vi "Config.vi"() -> ()   [LabVIEW 2020]
uses:
  Global_Variable/Global.vi
  Global_Variable/A180648.vi
  <vilib>/Utility/config.llb/NI_LVConfig.lvlib
  Libraries/S7/S7.lvlib
panel:
  in  "试验项目":cluster{"拉轴":bool, "卡簧":bool}
  in  "产品型号":string(combo)
  in  "删除":bool
  in  "确定":bool
  in  "添加":bool
  in  "退出":bool
  in  "更新":bool
  in  "选项卡控件":enum32{"产品参数"}(tab)
  in  "结果判定参数":string[][](table)=[["mm"], ["KN"], ["KN"], ["KN"], [""], [""], [""], [""], [""], [""], [""], [""]]
  in  "判定框参数":string[][](table)=[["mm"], ["KN"], ["mm"], ["KN"]]
  in  "坐标轴参数":string[][](table)=[[""], ["°/S"], ["°"], ["Nm"]]
  # "上转向轴组件压装"
types:
  T1 = typedef "NI_LVConfig.lvlib/Config Data RefNum.ctl" = refnum<k1>
  T2 = cluster{"[0]":cluster{string, dbl, dbl}, "[1]":cluster{string, dbl, dbl}, "[2]":cluster{string, dbl, dbl}, "[3]":cluster{string, dbl, dbl}}
  T3 = cluster{"第一段位移":cluster{"单位":string, "下限":dbl, "上限":dbl}, "第一段压力":cluster{"单位":string, "下限":dbl, "上限":dbl}, "第二段位移":cluster{"单位":string, "下限":dbl, "上限":dbl}, "第二段压力":cluster{"单位":string, "下限":dbl, "上限":dbl}}
  T4 = cluster{"[0]":cluster{string, dbl, dbl}, "[1]":cluster{string, dbl, dbl}, "[2]":cluster{string, dbl, dbl}, "[3]":cluster{string, dbl, dbl}, "[4]":cluster{string, dbl, dbl}}
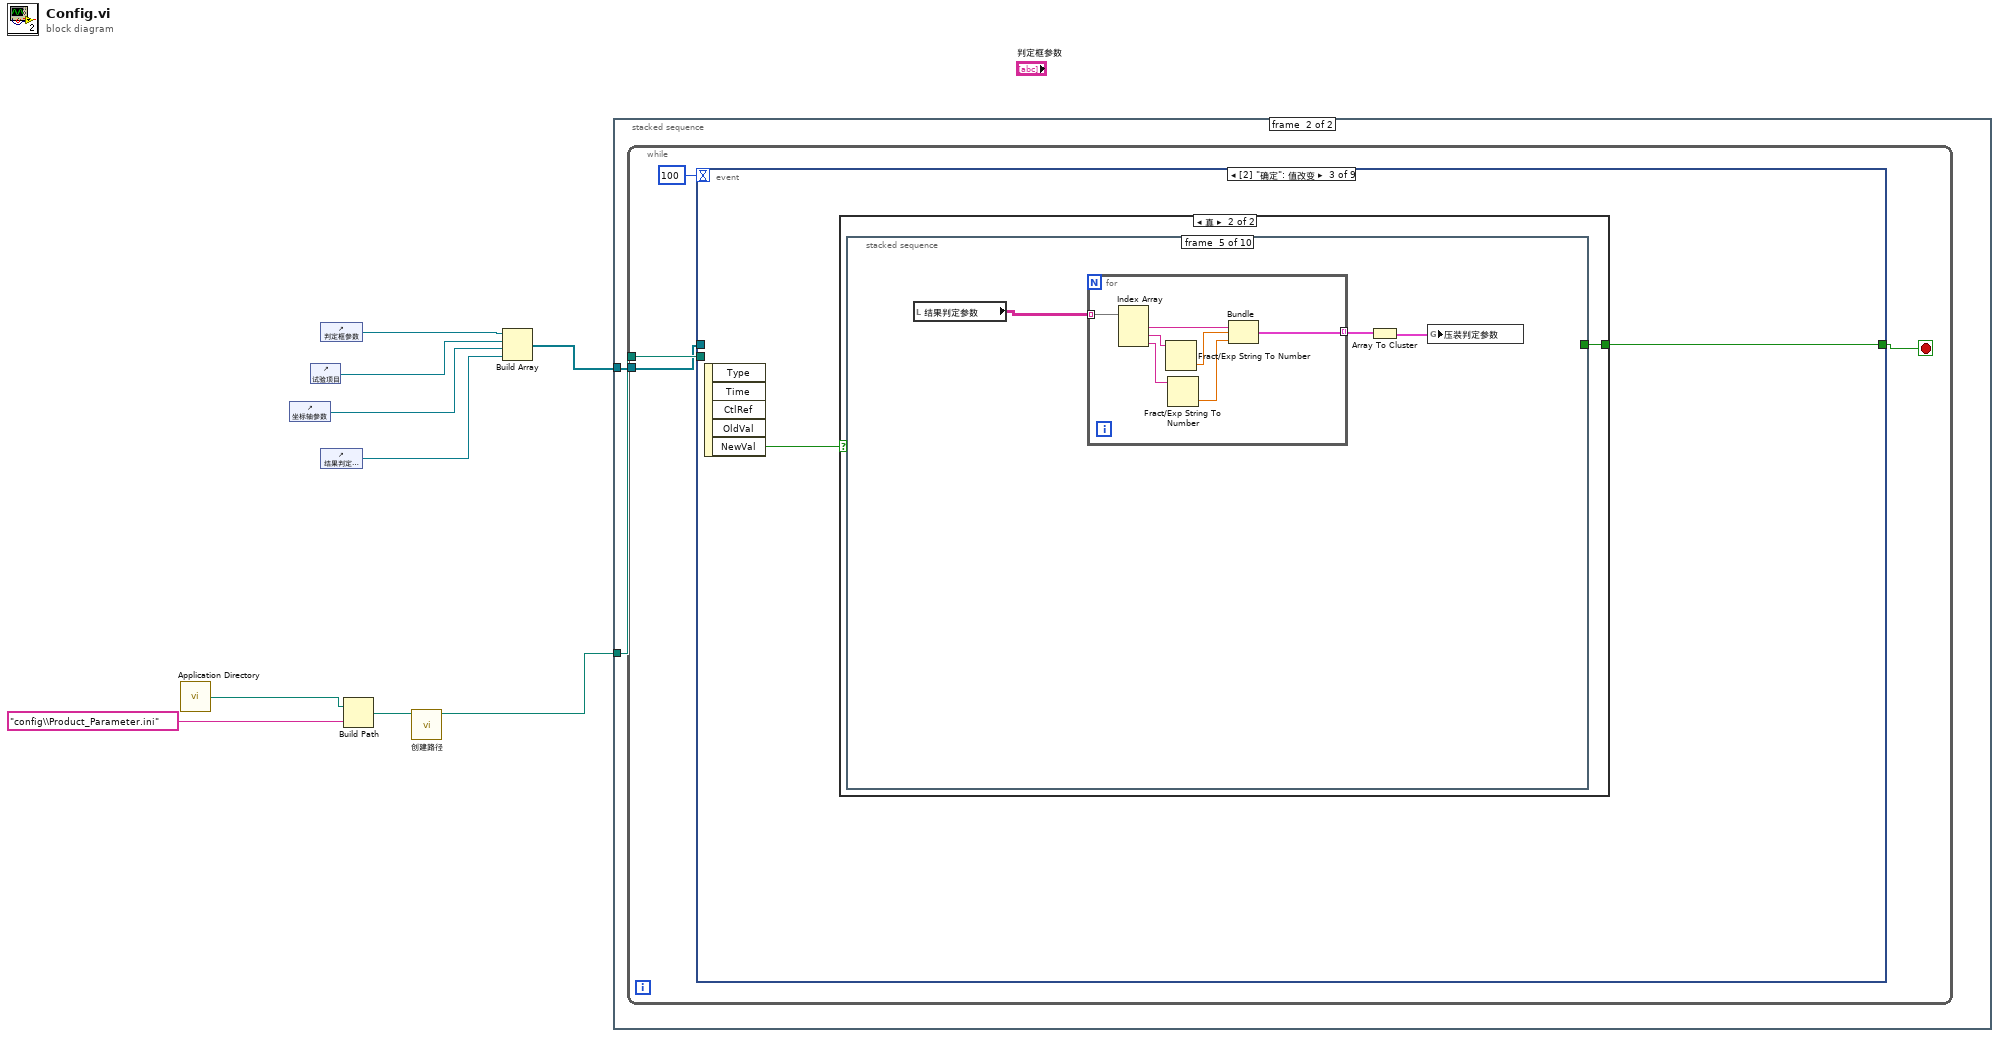
[diagram p0: block diagram]
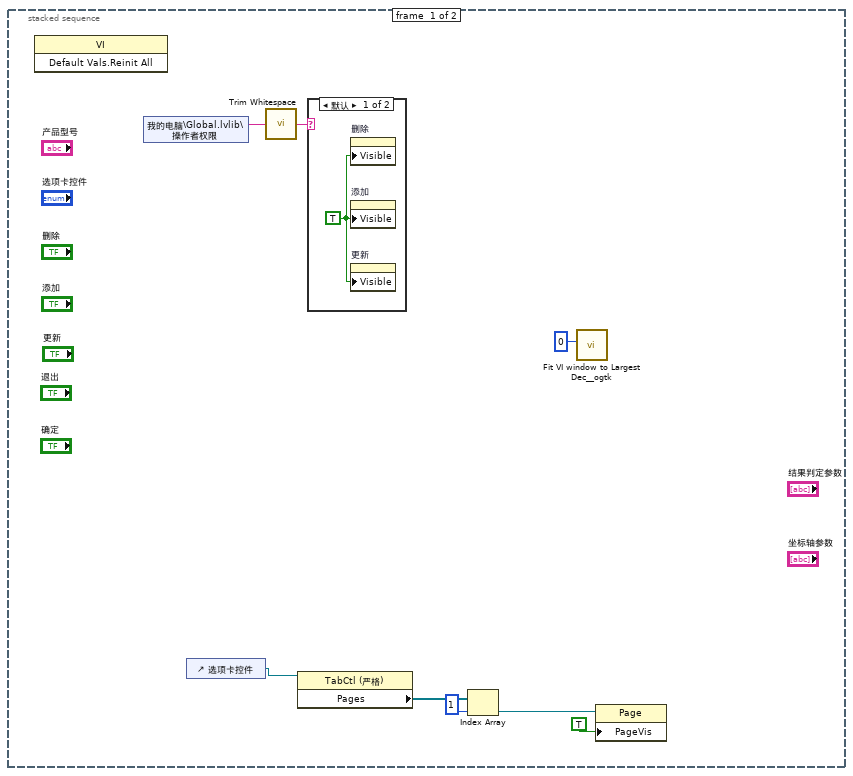
[diagram p2: hidden frame]
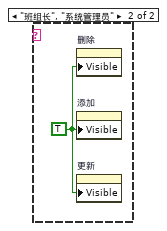
[diagram p3: hidden frame]
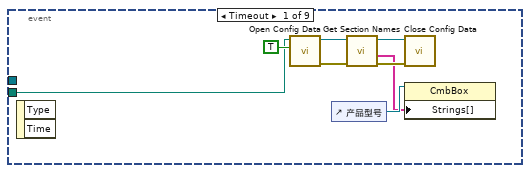
[diagram p4: hidden frame]
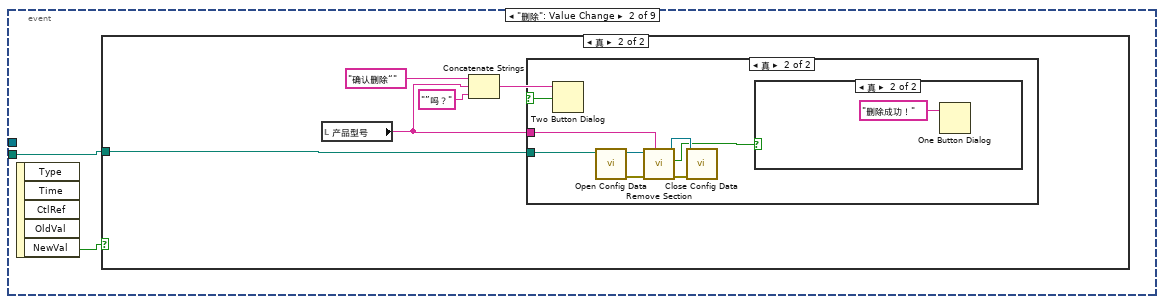
[diagram p5: hidden frame]
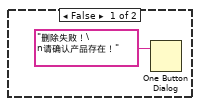
[diagram p8: hidden frame]
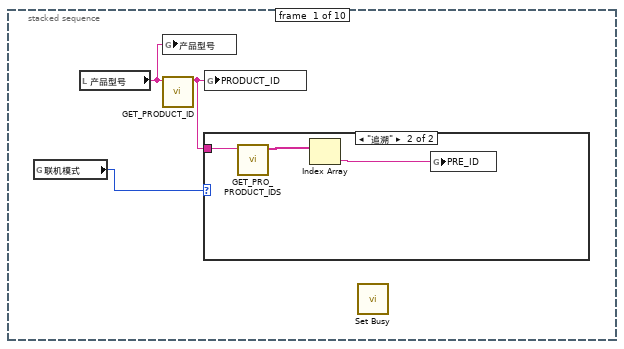
[diagram p10: hidden frame]
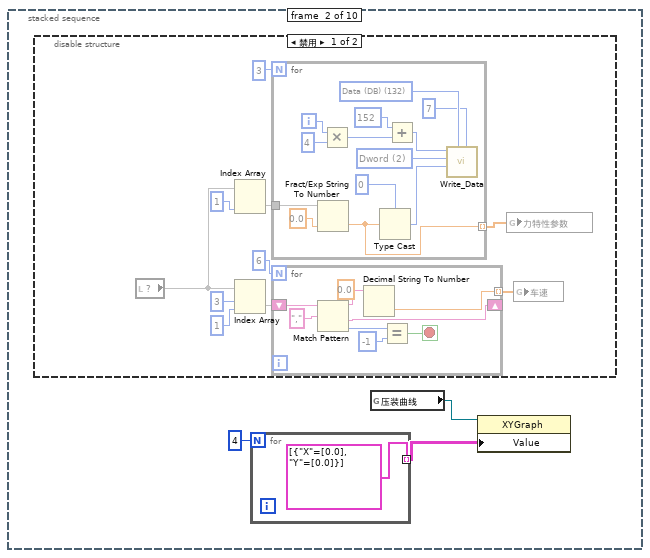
[diagram p12: hidden frame]
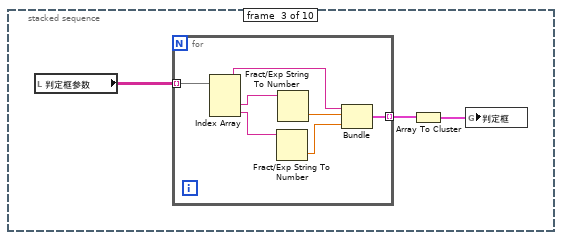
[diagram p14: hidden frame]
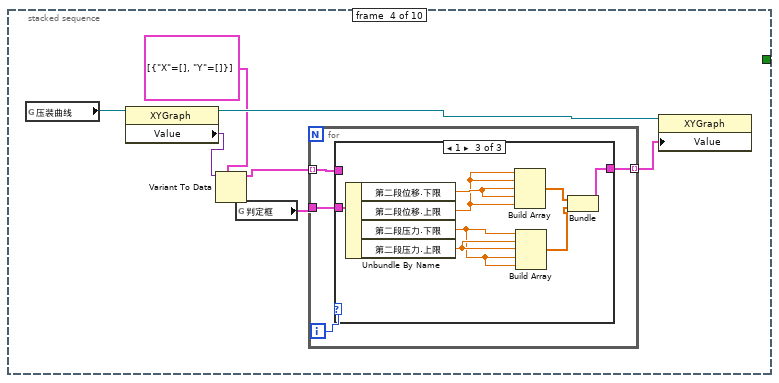
[diagram p15: hidden frame]
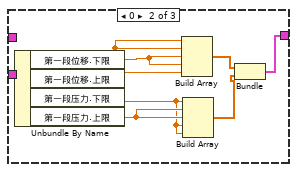
[diagram p17: hidden frame]
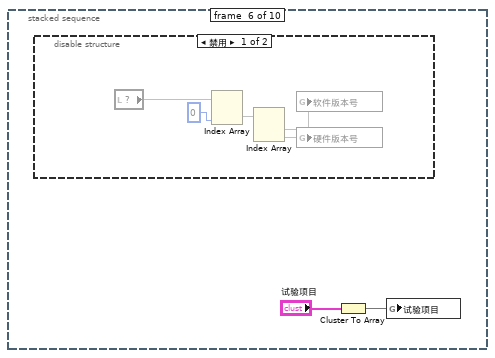
[diagram p18: hidden frame]
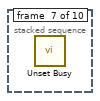
[diagram p20: hidden frame]
diagram:
  n1 = call <vilib>:"Application Directory.vi"() -> ("Application Directory"=w8:path)
  n2 = control-ref of="坐标轴参数"() -> (w3:refnum<vi>)
  n3 = control-ref of="试验项目"() -> (w4:refnum<vi>)
  n4 = control-ref of="判定框参数"() -> (w1:refnum<vi>)
  n5 = control-ref of="结果判定参数"() -> (w2:refnum<vi>)
  n6 = Build Path(base path=w8, name or relative path="config\\Product_Parameter.ini" ("名称或相对路径")) -> (appended path=w6:path)
  n7 = call "创建路径.vi"("path"=w6) -> ("path out"=w5:path)  [unwired: 9 in, 1 out]
  n8 = Build Array(w1, w4, w3, w2) -> (w9:refnum<vi>[])
  n9 = stacked-sequence {
    tunnel: w9 -> [_ w21]
    tunnel: w5 -> [_ w20]
    frame #0 {
      n10 = invoke class="VI" method="Default Vals.Reinit All"() -> ()  [unwired: 3 in, 3 out]
      n11 = shared-variable "我的电脑\\Global.lvlib\\操作者权限"() -> (w17:string)  [unwired: 1 in, 1 out]
      n12 = control-ref of="选项卡控件"() -> (w14:refnum<vi>)
      n13 = call <vilib>:"Trim Whitespace.vi"("string"=w17) -> ("trimmed string"=w16:string)  [unwired: 1 in]
      n14 = property class="TabCtl (严格)"(reference=w14) -> ("Pages"=w13:refnum<vi>[])  [unwired: 1 in, 2 out]
      n15 = case shown="默认" w16 {
        frame Default {
          w18 = TRUE ("可见")
          n16 = property on="删除" class="Bool (严格)"("Visible"=w18) -> ()  [unwired: 2 in, 2 out]
          n17 = property on="添加" class="Bool (严格)"("Visible"=w18) -> ()  [unwired: 2 in, 2 out]
          n18 = property on="更新" class="Bool (严格)"("Visible"=w18) -> ()  [unwired: 2 in, 2 out]
        }
        frame "班组长", "系统管理员" {
          w19 = TRUE ("可见")
          n19 = property on="删除" class="Bool (严格)"("Visible"=w19) -> ()  [unwired: 2 in, 2 out]
          n20 = property on="添加" class="Bool (严格)"("Visible"=w19) -> ()  [unwired: 2 in, 2 out]
          n21 = property on="更新" class="Bool (严格)"("Visible"=w19) -> ()  [unwired: 2 in, 2 out]
        }
      }
      n22 = Index Array(array=w13, index=1 ("索引")) -> (element=w12:refnum<vi>)
      n23 = call <userlib>:"Fit VI window to Largest Dec__ogtk.vi"("border spacing (2 px)"=0) -> ()  [unwired: 5 in, 2 out]
      n24 = property class="Page"(reference=w12, "PageVis"=TRUE ("选项卡可见")) -> ()  [unwired: 1 in, 2 out]
    }
    frame #1 {
      n25 = while {
        tunnel: w20 -> [w25]
        tunnel: w21 -> [w23]
        stop <- w24 stop-if-true
        n26 = event shown="[2] \"确定\": 值改变" {
          selector: _ -> [_ _ _ _ _ _ _ _ _]
          dyn-events: _ -> [_ _ _ _ _ _ _ _ _]
          timeout: 100 -> [_ _ _ _ _ _ _ _ _]
          tunnel: w25 -> [w28 w35 _ _ w160 w187 _ w211 _]
          tunnel: [_ _ w51 _ _ _ TRUE _ TRUE] -> w24
          tunnel: w23 -> [_ _ _ _ w161 w188 _ w210 _]
          event Timeout {
            n27 = event-data() -> ()  [unwired: 1 in, 2 out]
            n28 = call <vilib>:"Open Config Data.vi"("create file if necessary (T)"=TRUE, "configuration file path"=w28) -> ("error out"=w30:errorcluster, "refnum"=w29:T1)  [unwired: 7 in, 1 out]
            n29 = control-ref of="产品型号"() -> (w27:refnum<vi>)
            n30 = call <vilib>:"Get Section Names.vi"("error in (no error)"=w30, "refnum"=w29) -> ("error out"=w32:errorcluster, "section names"=w26:string[], "refnum out"=w31:T1)  [unwired: 7 in]
            n31 = call <vilib>:"Close Config Data.vi"("error in (no error)"=w32, "refnum"=w31) -> ()  [unwired: 8 in, 2 out]
            n32 = property on="属性节点" class="CmbBox"(reference=w27, "Strings[]"=w26) -> ()  [unwired: 1 in, 2 out]
          }
          event "删除": Value Change {
            n33 = event-data() -> ("NewVal"=w34:bool)  [unwired: 1 in, 4 out]
            n34 = case shown="真" w34 {
              tunnel: w35 -> [_ w37]
              frame False {
              }
              frame True {
                n35 = local read "产品型号"() -> (w36:string)
                n36 = Concatenate Strings("确认删除“", w36, "”吗？") -> (w39:string)
                n37 = Two Button Dialog(message=w39) -> (T button?=w38:bool)  [unwired: 2 in]
                n38 = case shown="真" w38 {
                  tunnel: w37 -> [_ w43]
                  tunnel: w36 -> [_ w42]
                  frame False {
                  }
                  frame True {
                    n39 = call <vilib>:"Open Config Data.vi"("configuration file path"=w43) -> ("error out"=w45:errorcluster, "refnum"=w48:T1)  [unwired: 8 in, 1 out]
                    n40 = call <vilib>:"Remove Section.vi"("section"=w42, "error in (no error)"=w45, "refnum"=w48) -> ("error out"=w47:errorcluster, "section exists?"=w44:bool, "refnum out"=w46:T1)  [unwired: 6 in]
                    n41 = call <vilib>:"Close Config Data.vi"("error in (no error)"=w47, "refnum"=w46) -> ()  [unwired: 8 in, 2 out]
                    n42 = case shown="真" w44 {
                      frame False {
                        n43 = One Button Dialog(message="删除失败！\n请确认产品存在！" ("消息")) -> ()  [unwired: 1 in, 1 out]
                      }
                      frame True {
                        n44 = One Button Dialog(message="删除成功！" ("消息")) -> ()  [unwired: 1 in, 1 out]
                      }
                    }
                  }
                }
              }
            }
          }
          event "确定": Value Change {
            n45 = event-data() -> ("NewVal"=w52:bool)  [unwired: 1 in, 4 out]
            n46 = case shown="真" w52 {
              tunnel: [_ w53] -> w51
              frame False {
              }
              frame True {
                n47 = stacked-sequence {
                  tunnel: [_ _ _ _ _ _ _ _ _ TRUE] -> w53
                  frame #0 {
                    n48 = global read "Global.vi" "联机模式"() -> (w54:enum16{"单机", "追溯"})
                    n49 = local read "产品型号"() -> (w56:string)
                    n50 = global write "Global.vi" "产品型号"(w56) -> ()
                    n51 = call "GET_PRODUCT_ID.vi"("PRODFUCT_NAME"=w56) -> ("PRODUCT_ID"=w55:string)  [unwired: 10 in]
                    n52 = case shown="\"追溯\"" w54 {
                      tunnel: w55 -> [_ w59]
                      frame "单机", Default {
                      }
                      frame "追溯" {
                        n53 = call "GET_PRO_PRODUCT_IDS.vi"("PRODUCT_ID"=w59) -> ("前序工位"=w58:string[])  [unwired: 10 in]
                        n54 = Index Array(array=w58) -> (element=w57:string)  [unwired: 1 in]
                        n55 = global write "追溯Global.vi" "PRE_ID"(w57) -> ()
                      }
                    }
                    n56 = global write "追溯Global.vi" "PRODUCT_ID"(w55) -> ()
                    n57 = call <vilib>:"Set Busy.vi"() -> ()  [unwired: 10 in, 2 out]
                  }
                  frame #1 {
                    n58 = disable-structure shown="禁用" {
                      frame Disabled {
                        n59 = local read item#-1() -> (w70)
                        n60 = Index Array(array=w70, index (col)=1 ("禁用的索引 (列)")) -> (element=w73)  [unwired: 1 in]
                        n61 = Index Array(array=w70, index (row)=3 ("索引 (行)"), index (col)=1 ("禁用的索引 (列)")) -> (element=w67)
                        n62 = for {
                          N: 3 -> [_]
                          tunnel: w73 -> [w91]
                          tunnel: [w83] -> w64 mode=indexing
                          i -> [w86]
                          w93 = u16 2 items=["byte", "word", "Dword"] ("数据类型")
                          w95 = u8 132 items=["I/O (P)"=128, "Input (I)"=129, "Output (Q)"=130, "Bit Memory (M)"=131, "Data (DB)"=132, "Instance Data (DI)"=133, "Local Data (L)"=134, "Predecessor Local Data (VL)"=135] ("寄存器类型")
                          n63 = Fract/Exp String To Number(string=w91, default (0 dbl)=sgl 0.0) -> (number=w83:sgl)  [unwired: 2 in, 1 out]
                          n64 = Multiply(x=w86, y=4) -> (x*y=w87:i32)
                          n65 = Type Cast(type=u32 0 ("写入地址"), x=w83) -> (*(type *) &x=w89:u32)
                          n66 = Add(x=u32 152 ("写入地址"), y=w87) -> (x+y=w84:u32)
                          n67 = call "Write_Data.vi"("DB #"=u16 7, "寄存器类型"=w95, "写入数据"=w89, "数据类型"=w93, "写入地址"=w84) -> ()  [unwired: 4 in, 3 out]
                        }
                        n68 = for {
                          N: 6 -> [_]
                          shift-right: [w80] -> _
                          shift-left: w67 -> [w82]
                          tunnel: [w76] -> w66 mode=indexing
                          stop <- w75 stop-if-true
                          n69 = Match Pattern(string=w82, regular expression="," ("正则表达式")) -> (before substring=w77:string, after substring=w80:string, offset past match=w79:i32)  [unwired: 1 in, 1 out]
                          n70 = Decimal String To Number(string=w77, default (0L)=sgl 0.0 ("默认(0 I32)")) -> (number=w76:sgl)  [unwired: 1 in, 1 out]
                          n71 = Equal?(x=w79, y=-1) -> (x = y?=w75:bool)
                        }
                        n72 = global write "A180648.vi" "力特性参数"(w64) -> ()
                        n73 = global write "A180648.vi" "车速"(w66) -> ()
                      }
                      frame Enabled {
                      }
                    }
                    n74 = for {
                      N: 4 -> [_]
                      tunnel: [cluster{"X":dbl[], "Y":dbl[]}[] [{"X"=[0.0], "Y"=[0.0]}]] -> w62 mode=indexing
                    }
                    n75 = global read "A180648.vi" "压装曲线"() -> (w60:refnum<vi>)
                    n76 = property class="XYGraph"(reference=w60, "Value"=w62) -> ()  [unwired: 1 in, 2 out]
                  }
                  frame #2 {
                    n77 = local read "判定框参数"() -> (w98:string[][])
                    n78 = for {
                      tunnel: w98 -> [w105] mode=indexing
                      tunnel: [w99] -> w97 mode=indexing
                      n79 = Index Array(array=w105) -> (element #1=w102:string, element #2=w104:string, element #3=w103:string)  [unwired: 3 in]
                      n80 = Fract/Exp String To Number(string=w103) -> (number=w100:dbl)  [unwired: 3 in, 1 out]
                      n81 = Fract/Exp String To Number(string=w104) -> (number=w101:dbl)  [unwired: 3 in, 1 out]
                      n82 = Bundle(w102, w101, w100) -> (w99:cluster{string, dbl, dbl})  [unwired: 1 in]
                    }
                    n83 = Array To Cluster(array=w97) -> (cluster=w96:T2)
                    n84 = global write "判定参数.vi" "判定框"(w96) -> ()
                  }
                  frame #3 {
                    n85 = global read "A180648.vi" "压装曲线"() -> (w112:refnum<vi>)
                    n86 = property class="XYGraph"(reference=w112) -> (reference out=w109:refnum<vi>, "Value"=w111:variant)  [unwired: 1 in, 1 out]
                    n87 = Variant To Data(type=cluster{"X":dbl[], "Y":dbl[]}[] [{"X"=[], "Y"=[]}], Variant=w111) -> (data=w110:cluster{"X":dbl[], "Y":dbl[]}[])  [unwired: 1 in, 1 out]
                    n88 = global read "判定参数.vi" "判定框"() -> (w106:T3)
                    n89 = for {
                      tunnel: w110 -> [w115] mode=indexing
                      tunnel: [w114] -> w107 mode=indexing
                      tunnel: w106 -> [w113]
                      i -> [w116]
                      n90 = case shown="1" w116 {
                        tunnel: w115 -> [w117 _ _]
                        tunnel: [w117 w120 w128] -> w114
                        tunnel: w113 -> [_ w125 w129]
                        frame Default {
                        }
                        frame 0 {
                          n91 = Unbundle By Name(w125) -> ("第一段位移.下限"=w124:dbl, "第一段位移.上限"=w123:dbl, "第一段压力.下限"=w118:dbl, "第一段压力.上限"=w119:dbl)
                          n92 = Build Array(w123, w123, w124, w124, w123) -> (w122:dbl[])
                          n93 = Build Array(w118, w119, w119, w118, w118) -> (w121:dbl[])
                          n94 = Bundle(w122, w121) -> (w120:cluster{dbl[], dbl[]})  [unwired: 1 in]
                        }
                        frame 1 {
                          n95 = Unbundle By Name(w129) -> ("第二段位移.下限"=w133:dbl, "第二段位移.上限"=w132:dbl, "第二段压力.下限"=w126:dbl, "第二段压力.上限"=w127:dbl)
                          n96 = Build Array(w132, w132, w133, w133, w132) -> (w131:dbl[])
                          n97 = Build Array(w126, w127, w127, w126, w126) -> (w130:dbl[])
                          n98 = Bundle(w131, w130) -> (w128:cluster{dbl[], dbl[]})  [unwired: 1 in]
                        }
                      }
                    }
                    n99 = property class="XYGraph"(reference=w109, "Value"=w107) -> ()  [unwired: 1 in, 2 out]
                  }
                  frame #4 {
                    n100 = local read "结果判定参数"() -> (w136:string[][])
                    n101 = for {
                      tunnel: w136 -> [w138] mode=indexing
                      tunnel: [w137] -> w134 mode=indexing
                      n102 = Index Array(array=w138) -> (element #1=w143:string, element #2=w142:string, element #3=w140:string)  [unwired: 3 in]
                      n103 = Fract/Exp String To Number(string=w142) -> (number=w141:dbl)  [unwired: 3 in, 1 out]
                      n104 = Fract/Exp String To Number(string=w140) -> (number=w139:dbl)  [unwired: 3 in, 1 out]
                      n105 = Bundle(w143, w141, w139) -> (w137:cluster{string, dbl, dbl})  [unwired: 1 in]
                    }
                    n106 = Array To Cluster(array=w134) -> (cluster=w135:T4)
                    n107 = global write "判定参数.vi" "压装判定参数"(w135) -> ()
                  }
                  frame #5 {
                    n108 = disable-structure shown="禁用" {
                      frame Disabled {
                        n109 = local read item#-1() -> (w150)
                        n110 = Index Array(array=w150, index (col)=0 ("禁用的索引 (列)")) -> (element=w148)  [unwired: 1 in]
                        n111 = Index Array(array=w148) -> (element #1=w147, element #2=w146)  [unwired: 2 in]
                        n112 = global write "Global.vi" "软件版本号"(w147) -> ()
                        n113 = global write "Global.vi" "硬件版本号"(w146) -> ()
                      }
                      frame Enabled {
                      }
                    }
                    n114 = Cluster To Array(cluster="试验项目") -> (array=w145:bool[])
                    n115 = global write "Global.vi" "试验项目"(w145) -> ()
                  }
                  frame #6 {
                    n116 = call <vilib>:"Unset Busy.vi"() -> ()  [unwired: 11 in, 1 out]
                  }
                  frame #7 {
                    n117 = global read "Global.vi" "更换产品"() -> (w152:refnum<vi>)
                    n118 = vi-ref "Auto.vi"() -> (w151:refnum<vi>)
                    n119 = property class="VIRef"(reference=w152, "Val(Sgnl)"=w151) -> ()  [unwired: 1 in, 2 out]
                  }
                  frame #8 {
                    w153 = 64 items=["None"=0, "Hand, Error, Stop"=16, "Question"=32, "Exclamation, Warning"=48, "Asterisk, Information"=64] ("icon")
                    w155 = "参数装载成功！" ("消息")
                    n120 = call "浮动通知.vi"("通知内容"=w155) -> ()  [unwired: 11 in]
                    n121 = call "信息框（标题、文本、图标）.vi"("icon"=w153, "caption"="参数加载", "text"=w155) -> ()  [unwired: 7 in, 2 out]
                  }
                  frame #9 {
                    n122 = control-ref of="本VI"() -> (w156:refnum<vi>)
                    n123 = invoke class="VI" method="FP.Close"(reference=w156) -> ()  [unwired: 2 in, 3 out]
                  }
                }
              }
            }
          }
          event "试验项目.卡簧": Value Change {
            n124 = event-data() -> ("NewVal"=w158:bool)  [unwired: 1 in, 5 out]
            n125 = case shown="真" w158 {
              frame False {
              }
              frame True {
                (unwired) FALSE ("值")
              }
            }
          }
          event "添加": Value Change {
            n126 = event-data() -> ("NewVal"=w159:bool)  [unwired: 1 in, 4 out]
            n127 = case shown="真" w159 {
              tunnel: w161 -> [_ w165]
              tunnel: w160 -> [_ w164]
              frame False {
              }
              frame True {
                n128 = call "产品添加提示：用户输入"() -> ("产品型号"=w162:string, "确定"=w163:bool)  [unwired: 17 in, 1 out]
                n129 = case shown="真" w163 {
                  tunnel: w165 -> [_ w168]
                  tunnel: w164 -> [_ w167]
                  tunnel: w162 -> [_ w166]
                  frame False {
                  }
                  frame True {
                    n130 = case shown="默认" w166 {
                      selector: w166 -> [_ w171]
                      tunnel: w168 -> [_ w174]
                      tunnel: w167 -> [_ w173]
                      frame "" {
                        n131 = One Button Dialog(message="产品名称不得为空!" ("text")) -> ()  [unwired: 1 in, 1 out]
                      }
                      frame Default {
                        n132 = property on="产品型号" class="CmbBox"() -> ("Strings[]"=w172:string[])  [unwired: 2 in, 2 out]
                        n133 = Search 1D Array(1D array=w172, element=w171) -> (index of element=w170:i32)  [unwired: 1 in]
                        n134 = case shown="-1" w170 {
                          tunnel: w174 -> [_ w178]
                          tunnel: w173 -> [_ w177]
                          tunnel: w171 -> [_ w176]
                          frame Default {
                            n135 = One Button Dialog(message="产品已存在！" ("消息")) -> ()  [unwired: 1 in, 1 out]
                          }
                          frame -1 {
                            n136 = stacked-sequence {
                              tunnel: w178 -> [w184 _]
                              tunnel: w177 -> [w183 _]
                              tunnel: w176 -> [w182 _]
                              frame #0 {
                                n137 = call <vilib>:"Set Busy.vi"() -> ("error out"=w180:errorcluster)  [unwired: 10 in, 1 out]
                                n138 = call "Read_Write INI File.vi"("Mode"=enum16{"Read", "Write"}."Write", "Section"=w182, "error in"=w180, "Filepath"=w183, "Ctl Refnum"=w184) -> ("error out"=w179:errorcluster)  [unwired: 6 in]
                                n139 = call <vilib>:"Unset Busy.vi"("error in (no error)"=w179) -> ()  [unwired: 10 in, 1 out]
                              }
                              frame #1 {
                                n140 = One Button Dialog(message="添加成功！" ("消息")) -> ()  [unwired: 1 in, 1 out]
                              }
                            }
                          }
                        }
                      }
                    }
                  }
                }
              }
            }
          }
          event "产品型号": Value Change {
            n141 = event-data() -> ("NewVal"=w186:string)  [unwired: 1 in, 4 out]
            n142 = stacked-sequence {
              tunnel: w188 -> [_ _ w192]
              tunnel: w187 -> [_ _ w191]
              tunnel: w186 -> [_ w190 _]
              frame #0 {
                n143 = control-ref of="本VI"() -> (w189:refnum<vi>)
                n144 = invoke class="VI" method="Default Vals.Reinit All"(reference=w189) -> ()  [unwired: 2 in, 3 out]
              }
              frame #1 {
                n145 = local write "产品型号"(w190) -> ()
              }
              frame #2 {
                n146 = disable-structure shown="启用" {
                  disable-tunnel: w192 -> [w194 w203]
                  disable-tunnel: w191 -> [w193 w204]
                  frame Disabled {
                    n147 = for {
                      tunnel: w194 -> [w197] mode=indexing
                      tunnel: w193 -> [w196]
                      n148 = local read "产品型号"() -> (w195:string)
                      n149 = call "Read_Write ParaINI File.vi"("Mode"=enum16{"Read", "Write"}."Read", "Section"=w195, "Filepath"=w196, "Ctl Refnum"=w197) -> ()  [unwired: 7 in, 1 out]
                    }
                  }
                  frame Enabled {
                    n150 = call <vilib>:"Set Busy.vi"() -> ("error out"=w199:errorcluster)  [unwired: 10 in, 1 out]
                    n151 = local read "产品型号"() -> (w202:string)
                    n152 = call "Read_Write INI File.vi"("Mode"=enum16{"Read", "Write"}."Read", "Section"=w202, "error in"=w199, "Filepath"=w204, "Ctl Refnum"=w203) -> ("error out"=w200:errorcluster)  [unwired: 6 in]
                    n153 = call <vilib>:"Unset Busy.vi"("error in (no error)"=w200) -> ()  [unwired: 10 in, 1 out]
                  }
                }
              }
            }
          }
          event "退出": Value Change {
            n154 = event-data() -> ()  [unwired: 1 in, 5 out]
            n155 = control-ref of="本VI"() -> (w207:refnum<vi>)
            n156 = invoke class="VI" method="FP.Close"(reference=w207) -> (reference out=w205:refnum<vi>, error out=w206:errorcluster)  [unwired: 2 in, 1 out]
            n157 = Close Reference(reference=w205, error in (no error)=w206) -> ()  [unwired: 1 out]
          }
          event "更新": Value Change {
            n158 = event-data() -> ("NewVal"=w209:bool)  [unwired: 1 in, 4 out]
            n159 = case shown="真" w209 {
              tunnel: w211 -> [_ w214]
              tunnel: w210 -> [_ w213]
              frame False {
              }
              frame True {
                n160 = disable-structure shown="启用" {
                  disable-tunnel: w214 -> [w217 w228]
                  disable-tunnel: w213 -> [w216 w223]
                  disable-tunnel: [w215 w225] -> w212
                  frame Disabled {
                    n161 = for {
                      tunnel: w217 -> [w220]
                      tunnel: w216 -> [w219] mode=indexing
                      tunnel: [w218] -> w215
                      n162 = local read "产品型号"() -> (w222:string)
                      n163 = call "Read_Write ParaINI File.vi"("Mode"=enum16{"Read", "Write"}."Write", "Section"=w222, "Filepath"=w220, "Ctl Refnum"=w219) -> ("error out"=w218:errorcluster)  [unwired: 7 in]
                    }
                  }
                  frame Enabled {
                    n164 = call <vilib>:"Set Busy.vi"() -> ("error out"=w224:errorcluster)  [unwired: 10 in, 1 out]
                    n165 = local read "产品型号"() -> (w227:string)
                    n166 = call "Read_Write INI File.vi"("Mode"=enum16{"Read", "Write"}."Write", "Section"=w227, "error in"=w224, "Filepath"=w228, "Ctl Refnum"=w223) -> ("error out"=w225:errorcluster)  [unwired: 6 in]
                  }
                }
                n167 = case shown="无错误" w212 {
                  frame No Error {
                    n168 = call <vilib>:"Unset Busy.vi"() -> ()  [unwired: 11 in, 1 out]
                    n169 = Wait (ms)(milliseconds to wait=u32 500 ("等待时间（毫秒）")) -> ()  [unwired: 1 out]
                    n170 = One Button Dialog(message="更新成功！" ("通知内容")) -> ()  [unwired: 1 in, 1 out]
                  }
                  frame Error {
                    n171 = Wait (ms)(milliseconds to wait=u32 500 ("等待时间（毫秒）")) -> ()  [unwired: 1 out]
                    n172 = call "浮动通知.vi"("通知内容"="更新失败！") -> ()  [unwired: 11 in]
                  }
                }
              }
            }
          }
          event Panel Close {
            n173 = event-data() -> ()  [unwired: 1 in, 3 out]
          }
        }
      }
    }
  }
